vi "Stop Core.vi"(10 "final error code":i32, 11 "Dual Fan in":refnum<class "Dual Fan.lvclass">) -> (3 "Dual Fan out":refnum<class "Dual Fan.lvclass">)   [LabVIEW 2012, in "Dual Fan.lvlib" / "Dual Fan.lvclass"]
doc: "(<B>Filename</B>: Actor Framework.lvlib:Actor.lvclass:Stop Core.vi)\n\nDefines what the actor does before it stops. Use the <B>final error code</B> input to determine whether the actor shut down in response to an error.\n\nBy default, this method does nothing. A descendant class may override it to define behavior, such as shutting down any processes the actor initiated in its override of the Actor Core method."
uses:
  Dual Fan.lvclass
  Timed Loop Controller/Timed Loop Controller/Timed Loop Controller.lvclass
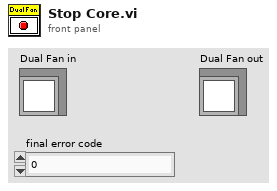
[diagram p1: front panel]
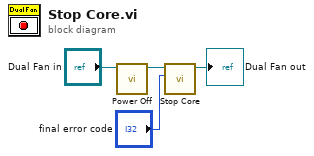
[diagram p0: block diagram]
diagram:
  n1 = call "Power Off.vi"("Dual Fan in"="Dual Fan in") -> ("Dual Fan out"=w1:refnum<class "Dual Fan.lvclass">)  [unwired: 9 in, 1 out]
  n2 = call-parent "Stop Core.vi"("final error code"="final error code", "Actor in"=w1) -> ("Actor out"=→"Dual Fan out":refnum<class "Dual Fan.lvclass">)  [unwired: 9 in]
